vi "Tutorial1.vi"() -> ()   [LabVIEW 2021]
uses:
  C:/TwinCAT/AdsApi/.NET/v4.0.30319/TwinCAT.Ads.dll
  TwinCAT/AdsApi/.NET/v4.0.30319/TwinCAT.Ads.dll
panel:
  in  "?":bool
  in  "Start Motor":bool
  in  "Stop Motor":bool
  out "Moto Run":bool
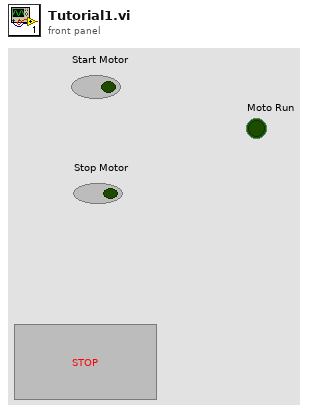
[diagram p1: front panel]
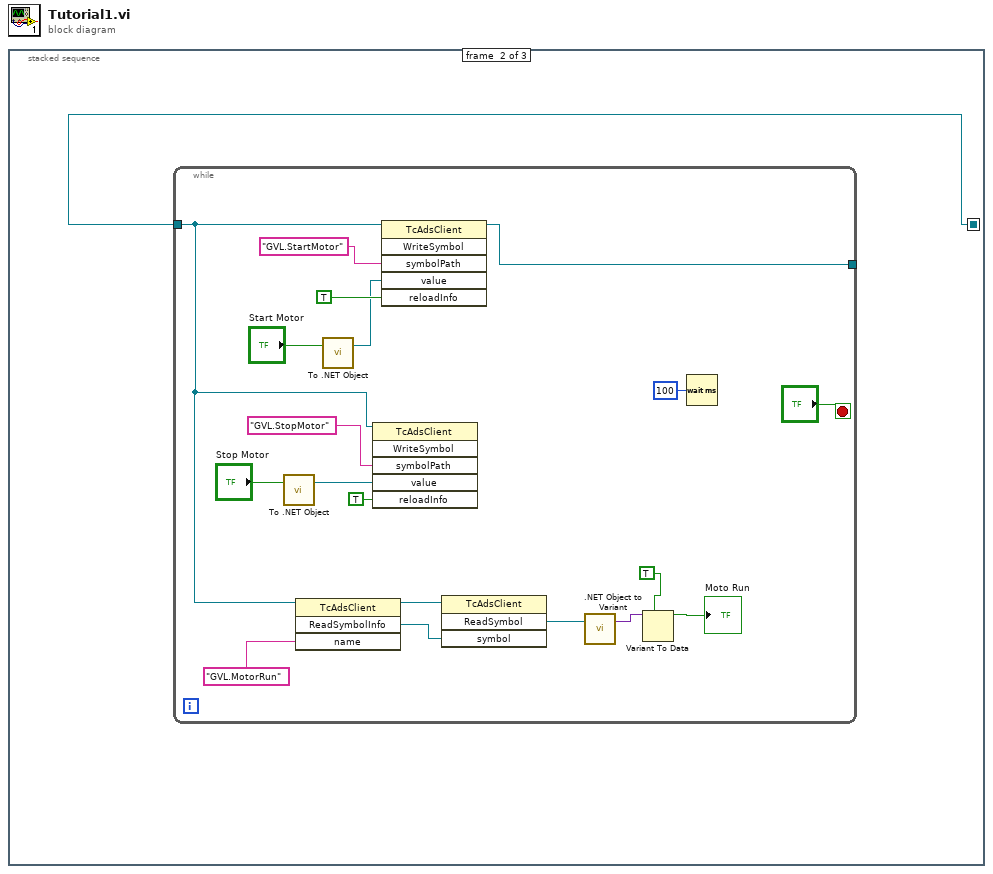
[diagram p0: block diagram]
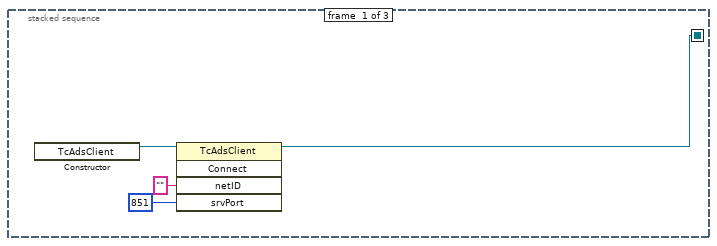
[diagram p2: hidden frame]
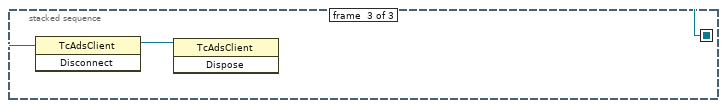
[diagram p3: hidden frame]
diagram:
  n1 = stacked-sequence {
    seq-local: [w1 _ _] -> [_ w5 w25]
    frame #0 {
      n2 = constructor class="TcAdsClient"() -> (reference out=w4:refnum<k24>)  [unwired: 3 in, 2 out]
      n3 = invoke class="TcAdsClient" method="Connect"(reference=w4, "netID"="", "srvPort"=851) -> (reference out=w1:refnum<k24>)  [unwired: 2 in, 4 out]
    }
    frame #1 {
      n4 = while {
        tunnel: [w7] -> _
        tunnel: w5 -> [w6]
        stop <- "?" stop-if-true
        n5 = call <vilib>:"To .NET Object.vi"("anything"="Stop Motor") -> (".NET object"=w17:refnum<k24>)  [unwired: 1 in, 1 out]
        n6 = invoke class="TcAdsClient" method="ReadSymbolInfo"(reference=w6, "name"="GVL.MotorRun" ("symbolPath")) -> (reference out=w12:refnum<k24>, "ReadSymbolInfo"=w13:refnum<k24>)  [unwired: 2 in, 2 out]
        n7 = call <vilib>:"To .NET Object.vi"("anything"="Start Motor") -> (".NET object"=w19:refnum<k24>)  [unwired: 1 in, 1 out]
        n8 = invoke class="TcAdsClient" method="WriteSymbol"(reference=w6, "symbolPath"="GVL.StopMotor", "value"=w17, "reloadInfo"=TRUE) -> ()  [unwired: 2 in, 6 out]
        n9 = invoke class="TcAdsClient" method="WriteSymbol"(reference=w6, "symbolPath"="GVL.StartMotor", "value"=w19, "reloadInfo"=TRUE) -> (reference out=w7:refnum<k24>)  [unwired: 2 in, 5 out]
        n10 = invoke class="TcAdsClient" method="ReadSymbol"(reference=w12, "symbol"=w13) -> ("ReadSymbol"=w11:refnum<k24>)  [unwired: 2 in, 3 out]
        n11 = call <vilib>:".NET Object to Variant.vi"(".NET object"=w11) -> ("variant"=w10:variant)  [unwired: 1 in, 1 out]
        n12 = Variant To Data(type=TRUE, Variant=w10) -> (data=→"Moto Run":bool)  [unwired: 1 in, 1 out]
        n13 = Wait (ms)(milliseconds to wait=u32 100) -> ()  [unwired: 1 out]
      }
    }
    frame #2 {
      n14 = invoke class="TcAdsClient" method="Disconnect"(reference=w25) -> (reference out=w26:refnum<k24>)  [unwired: 2 in, 2 out]
      n15 = invoke class="TcAdsClient" method="Dispose"(reference=w26) -> ()  [unwired: 2 in, 3 out]
    }
  }
